vi "REceptorUSART.vi"() -> ()   [LabVIEW 2015]
uses:
  <vilib>/Instr/_visa.llb/Select Event Type.ctl
  <vilib>/Instr/_visa.llb/VISA Configure Serial Port (Instr).vi
panel:
  out "Humedades y Potencia lumínica":cluster{"f":dbl, "f":dbl, "f":i32}(graph)
  in  "Plot Humedad Tierra":bool
  in  "Plot Potencia Luminica":bool
  in  "Plot Humedad Relativa":bool
  out "Humedad Relativa %":dbl(knob) scale=0.0..100.0
  out "Humedad Tierra %":dbl(knob) scale=0.0..100.0
  out "Potencia Lumínica %":dbl(knob) scale=0.0..100.0
  in  "Plot MCP9808":bool
  in  "Plot Temp DHT22":bool
  in  "Plot Analog Temp":bool
  out "Termometro I2C MCP9808":dbl(slide) scale=-20.0..50.0
  out "Temp Analog":i16(slide) caption="Thermometer" scale=-20.0..50.0
  out "Temp Digital":i16(slide) caption="Thermometer" scale=-20.0..50.0
  out "Temperaturas":cluster{i32, "f":i32, "f":i32}(graph)
  in  "Solicitar Muestras":bool
  out "ON":bool
  in  "stop":bool
  out "read buffer":string
  in  "PORT COM IMPUT":refnum<visa-resource-name>
  # "DHT22 Sensor"
  # "Control Panel"
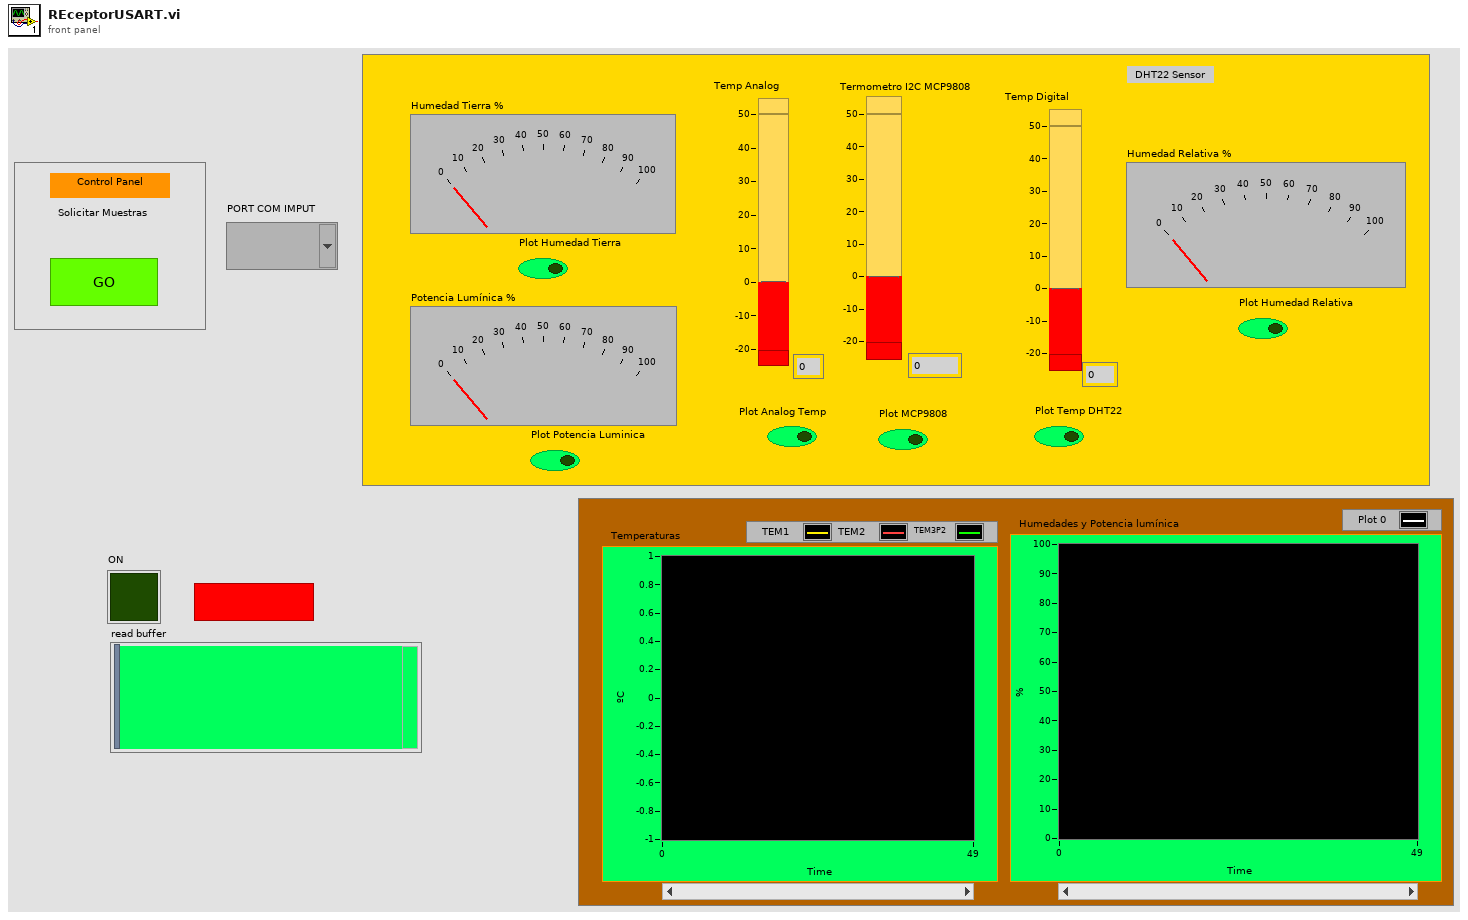
[diagram p1: front panel]
types:
  T1 = typedef "Select Event Type.ctl" = u32
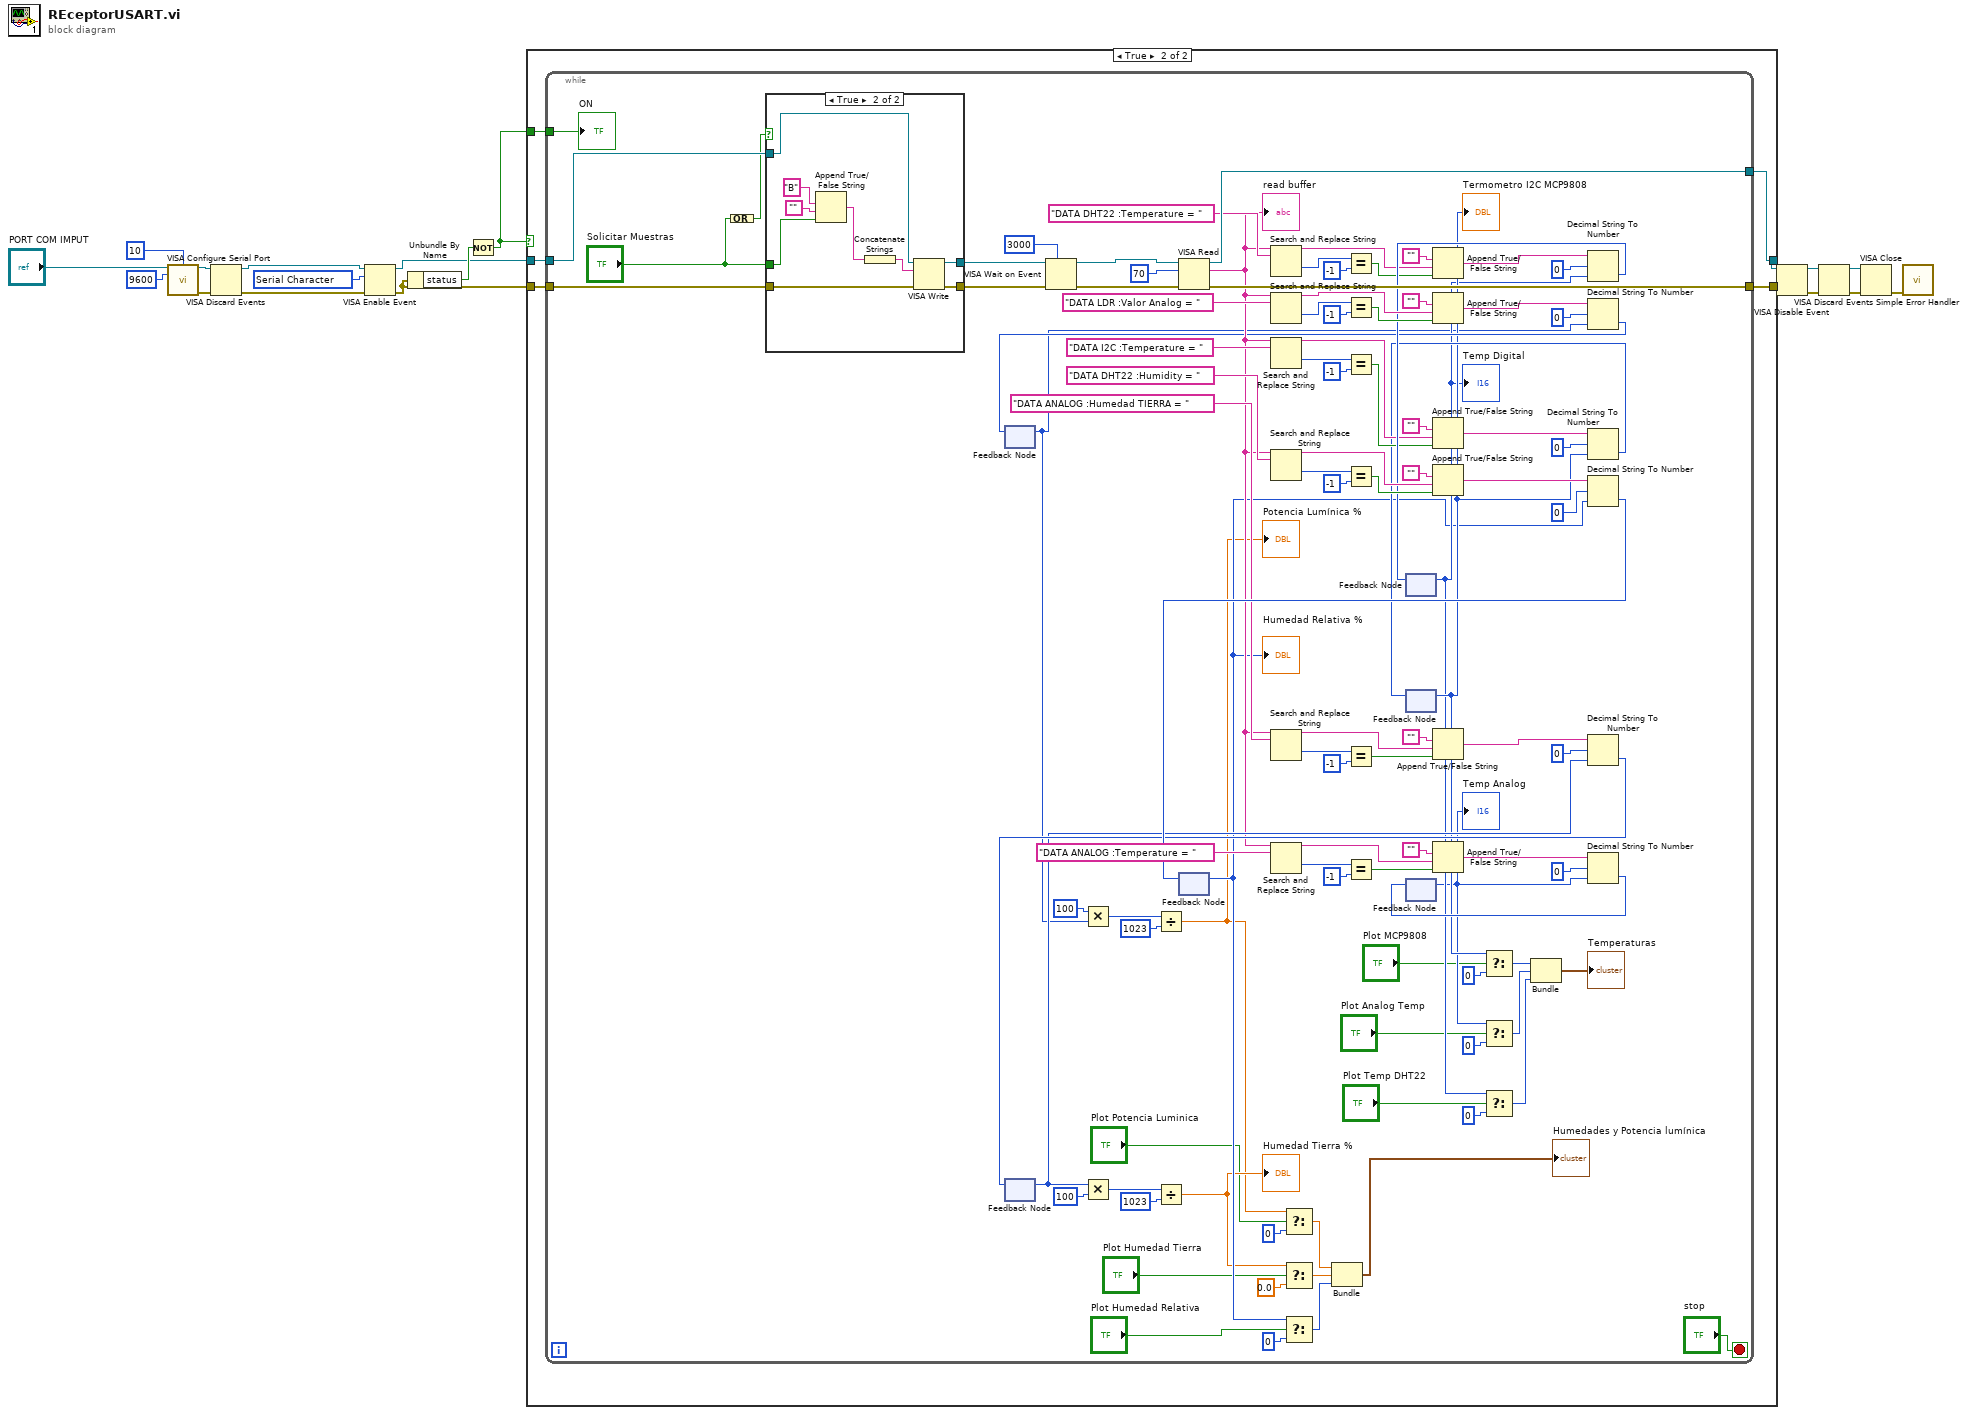
[diagram p0: block diagram]
diagram:
  w16 = T1 1073684533 items=["Service Request"=1073684491, "Trigger"=3221168138, "Clear"=1073684493, "VXI Signal"=1073684512, "VXI/VME Interrupt"=3221168161, "VXI/VME Sysfail"=1073684509, "VXI/VME Sysreset"=1073684510, "GPIB CIC"=1073684498, "GPIB Talk"=1073684499, "GPIB Listen"=1073684500, "PXI Interrupt"=1073684514, "Serial Break"=1073684515, "Serial TermChar"=1073684516, "Serial CTS"=1073684521, "Serial DSR"=1073684522, "Serial DCD"=1073684524, "Serial RI"=1073684526, "Serial Character"=1073684533, "USB Interrupt"=1073684535, "All Enabled"=1073709055] ("Event Type")
  n1 = call-poly "VISA Configure Serial Port"("VISA resource name"="PORT COM IMPUT", "termination char\n(0xA = '\\n' = LF)"=u8 10 ("termination char\n(0xA = '\\n' = LF)"), "baud rate (9600)"=u32 9600) -> ("VISA resource name out"=w4:refnum<visa-resource-name>, "error out"=w3:errorcluster)  [unwired: 11 in]
  n2 = VISA Discard Events(8:w3, 11:w4) -> (0:w17:errorcluster, 3:w18:refnum<visa-resource-name>)  [unwired: 2 in]
  n3 = VISA Enable Event(8:w17, 10:w16, 11:w18) -> (0:w1:errorcluster, 3:w2:refnum<visa-resource-name>)  [unwired: 1 in]
  n4 = Unbundle By Name(w1) -> ("status"=w15:bool)
  n5 = Not(x=w15) -> (.not. x?=w8:bool)
  n6 = case shown="True" w8 {
    tunnel: w1 -> [w21 w26]
    tunnel: w2 -> [w20 w25]
    tunnel: w8 -> [_ w24]
    tunnel: [w21 w22] -> w10
    tunnel: [w20 w23] -> w9
    frame False {
    }
    frame True {
      n7 = while {
        tunnel: w26 -> [w119]
        tunnel: w25 -> [w118]
        tunnel: w24 -> [w124]
        tunnel: [w126] -> w23
        tunnel: [w125] -> w22
        stop <- "stop" stop-if-true
        n8 = Compound Arithmetic op=OR("Solicitar Muestras") -> (w115:bool)
        n9 = case shown="True" w115 {
          tunnel: w118 -> [w131 w140]
          tunnel: w119 -> [w130 w139]
          tunnel: [w131 w138] -> w121
          tunnel: [w130 w137] -> w120
          tunnel: "Solicitar Muestras" -> [_ w134]
          frame False {
          }
          frame True {
            n10 = Append True/False String(1:w134, 2:"", 3:"B") -> (0:w135:string)  [unwired: 1 in]
            n11 = Concatenate Strings(w135) -> (w136:string)
            n12 = VISA Write(VISA resource name=w140, write buffer=w136, error in (no error)=w139) -> (VISA resource name out=w138:refnum<visa-resource-name>, error out=w137:errorcluster)  [unwired: 1 out]
          }
        }
        n13 = feedback #1() -> (w41:i32)  [unwired: 1 in]
        n14 = feedback #2() -> (w71:i32)  [unwired: 1 in]
        n15 = VISA Wait on Event(7:u32 3000 ("timeout (0)"), 8:w120, 11:w121) -> (0:w129:errorcluster, 3:w128:refnum<visa-resource-name>)  [unwired: 2 in, 2 out]
        n16 = Multiply(x=100 ("y"), y=w41) -> (x*y=w43:i32)
        n17 = Multiply(x=w71, y=100) -> (x*y=w70:i32)
        n18 = Divide(x=w43, y=1023) -> (x/y=w33:dbl)
        "Potencia Lumínica %" <- w33
        n19 = Divide(x=w70, y=1023) -> (x/y=w34:dbl)
        "Humedad Tierra %" <- w34
        n20 = VISA Read(VISA resource name=w128, byte count=u32 70, error in (no error)=w129) -> (VISA resource name out=w126:refnum<visa-resource-name>, read buffer=w58:string, error out=w125:errorcluster)  [unwired: 1 out]
        "read buffer" <- w58
        n21 = feedback #3() -> (w35:i32)  [unwired: 1 in]
        "Humedad Relativa %" <- w35
        n22 = Search and Replace String(input string=w58, search string="DATA DHT22 :Temperature = ") -> (result string=w85:string, offset past replacement=w87:i32)  [unwired: 6 in, 2 out]
        n23 = Search and Replace String(input string=w58, search string="DATA LDR :Valor Analog = ") -> (result string=w108:string, offset past replacement=w110:i32)  [unwired: 6 in, 2 out]
        n24 = Search and Replace String(input string=w58, search string="DATA I2C :Temperature = ") -> (result string=w64:string, offset past replacement=w66:i32)  [unwired: 6 in, 2 out]
        n25 = Search and Replace String(input string=w58, search string="DATA DHT22 :Humidity = ") -> (result string=w102:string, offset past replacement=w104:i32)  [unwired: 6 in, 2 out]
        n26 = Search and Replace String(input string=w58, search string="DATA ANALOG :Humedad TIERRA = ") -> (result string=w77:string, offset past replacement=w79:i32)  [unwired: 6 in, 2 out]
        n27 = Search and Replace String(input string=w58, search string="DATA ANALOG :Temperature = ") -> (result string=w94:string, offset past replacement=w96:i32)  [unwired: 6 in, 2 out]
        n28 = Select(t=w33, s="Plot Potencia Luminica", f=0) -> (s? t:f=w36:dbl)
        n29 = Select(t=w34, s="Plot Humedad Tierra", f=0.0) -> (s? t:f=w39:dbl)
        n30 = Select(t=w35, s="Plot Humedad Relativa", f=0) -> (s? t:f=w38:i32)
        n31 = Bundle("f"=w36, "f"=w39, "f"=w38) -> (→"Humedades y Potencia lumínica":cluster{"f":dbl, "f":dbl, "f":i32})  [unwired: 1 in]
        n32 = Equal?(x=w87, y=-1) -> (x = y?=w84:bool)
        n33 = Equal?(x=w110, y=-1) -> (x = y?=w106:bool)
        n34 = Equal?(x=w66, y=-1) -> (x = y?=w63:bool)
        n35 = Equal?(x=w104, y=-1) -> (x = y?=w100:bool)
        n36 = Equal?(x=w79, y=-1) -> (x = y?=w76:bool)
        n37 = Equal?(x=w96, y=-1) -> (x = y?=w92:bool)
        n38 = feedback #4() -> (w51:i32)  [unwired: 1 in]
        "Temp Digital" <- w51
        n39 = feedback #5() -> (w54:i32)  [unwired: 1 in]
        "Termometro I2C MCP9808" <- w54
        n40 = feedback #6() -> (w50:i32)  [unwired: 1 in]
        "Temp Analog" <- w50
        n41 = Append True/False String(1:w84, 2:w85, 3:"") -> (0:w81:string)  [unwired: 1 in]
        n42 = Append True/False String(1:w106, 2:w108, 3:"") -> (0:w89:string)  [unwired: 1 in]
        n43 = Append True/False String(1:w63, 2:w64, 3:"") -> (0:w62:string)  [unwired: 1 in]
        n44 = Append True/False String(1:w100, 2:w102, 3:"") -> (0:w99:string)  [unwired: 1 in]
        n45 = Append True/False String(1:w76, 2:w77, 3:"") -> (0:w75:string)  [unwired: 1 in]
        n46 = Append True/False String(1:w92, 2:w94, 3:"") -> (0:w90:string)  [unwired: 1 in]
        n47 = Select(t=w54, s="Plot MCP9808", f=0) -> (s? t:f=w55:i32)
        n48 = Select(t=w50, s="Plot Analog Temp", f=0) -> (s? t:f=w53:i32)
        n49 = Select(t=w51, s="Plot Temp DHT22", f=0) -> (s? t:f=w52:i32)
        n50 = Bundle("f"=w55, "f"=w53, "f"=w52) -> (→"Temperaturas":cluster{"f":i32, "f":i32, "f":i32})  [unwired: 1 in]
        n51 = Decimal String To Number(string=w81, offset=0, default (0L)=w51) -> (number=w97:i32)  [unwired: 1 out]
        n52 = feedback-in #4(w97) -> ()
        n53 = Decimal String To Number(string=w89, offset=0, default (0L)=w41) -> (number=w57:i32)  [unwired: 1 out]
        n54 = feedback-in #1(w57) -> ()
        n55 = Decimal String To Number(string=w62, offset=0, default (0L)=w54) -> (number=w60:i32)  [unwired: 1 out]
        n56 = feedback-in #5(w60) -> ()
        n57 = Decimal String To Number(string=w99, offset=0, default (0L)=w35) -> (number=w98:i32)  [unwired: 1 out]
        n58 = feedback-in #3(w98) -> ()
        n59 = Decimal String To Number(string=w75, offset=0, default (0L)=w71) -> (number=w73:i32)  [unwired: 1 out]
        n60 = feedback-in #2(w73) -> ()
        n61 = Decimal String To Number(string=w90, offset=0, default (0L)=w50) -> (number=w88:i32)  [unwired: 1 out]
        n62 = feedback-in #6(w88) -> ()
        "ON" <- w124
      }
    }
  }
  n63 = VISA Disable Event(8:w10, 11:w9) -> (0:w11:errorcluster, 3:w12:refnum<visa-resource-name>)  [unwired: 2 in]
  n64 = VISA Discard Events(8:w11, 11:w12) -> (0:w14:errorcluster, 3:w13:refnum<visa-resource-name>)  [unwired: 2 in]
  n65 = VISA Close(VISA resource name=w13, error in (no error)=w14) -> (error out=w6:errorcluster)
  n66 = call <vilib>:"Simple Error Handler.vi"("error in (no error)"=w6) -> ()  [unwired: 1 in, 8 out]
